vi "setOnTheFlySpeed.vi"(0 "ACESDEController in":refnum<class "ACESDEController.lvclass">, 2 "axis (nc - for use only with multi-axis applications)":T1, 3 "speed":i32, 5 "error in (no error)":errorcluster) -> (14 "ACESDEController out":refnum<class "ACESDEController.lvclass">, 17 "success?":bool, 18 "response":string, 19 "error out":errorcluster)   [LabVIEW 2013, in "classes.lvlib" / "ACESDEController.lvclass"]
uses:
  ACESDEController.lvclass
  axis.ctl
  _Controller.lvclass
  common.lvlib
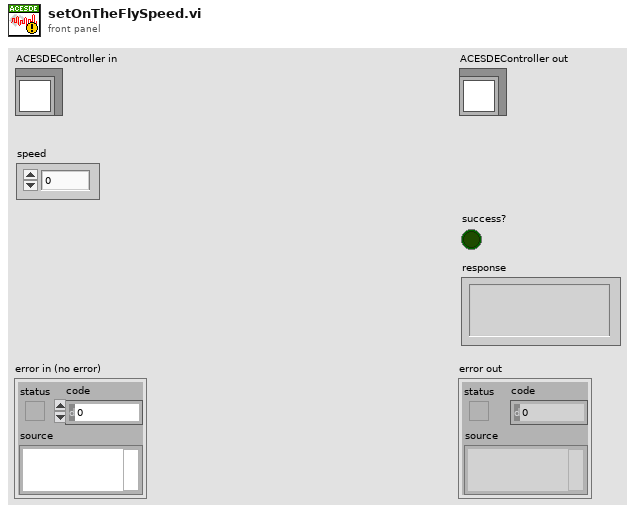
[diagram p1: front panel]
types:
  T1 = typedef "common.lvlib/axis.ctl" = enum16{"X", "Y", "Z", "U"}
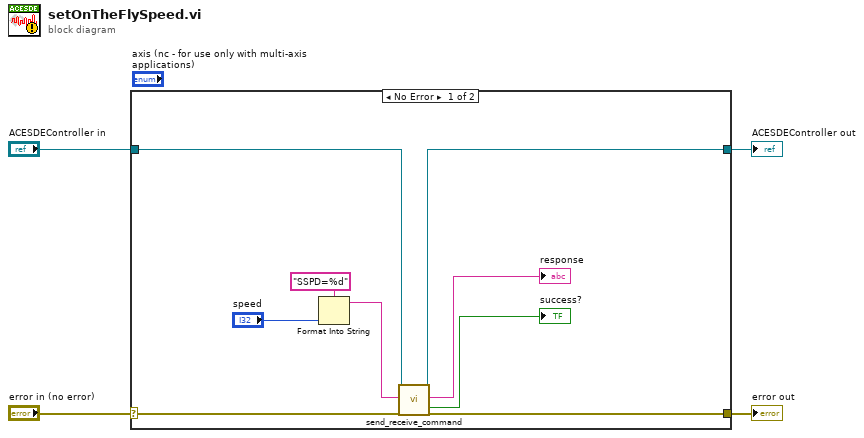
[diagram p0: block diagram]
diagram:
  n1 = case shown="No Error" "error in (no error)" {
    selector: "error in (no error)" -> [w11 w15]
    tunnel: [w10 w15] -> w3
    tunnel: [w8 w14] -> w1
    tunnel: "ACESDEController in" -> [w9 w14]
    frame No Error {
      n2 = Format Into String(format string="SSPD=%d", "speed") -> (resulting string=w5:string)  [unwired: 2 in, 1 out]
      n3 = call "send_receive_command.vi"("reference (in)"=w9, "ASCII Command (in)"=w5, "error in (no error)"=w11) -> ("reference (out)"=w8:refnum<class "ACESDEController.lvclass">, "response (out)"=→"response":string, "success?"=→"success?":bool, "error out"=w10:errorcluster)  [unwired: 12 in, 1 out]
    }
    frame Error {
    }
  }
  "error out" <- w3
  "ACESDEController out" <- w1
